vi "Convert I2C Messages & Buffer.vi"(8 "error in (no error)":errorcluster, 11 "Data":u8[](array[numeric])) -> (0 "error out":errorcluster)   [LabVIEW 2025, in "I2C Bus Monitor UI.lvlib"]
uses:
  I2C Bus Monitor UI.lvlib
  Table Buffer - Enqueue.vi
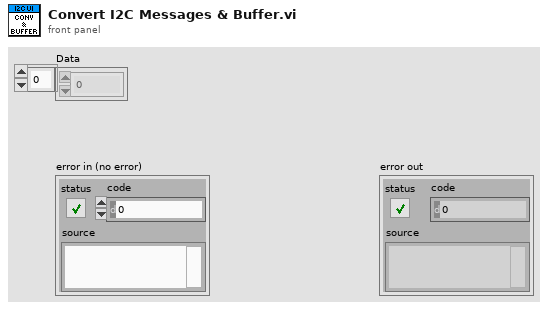
[diagram p1: front panel]
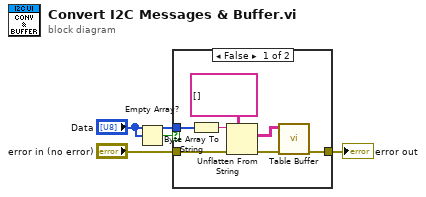
[diagram p0: block diagram]
diagram:
  n1 = Empty Array?(array="Data") -> (empty?=w2:bool)
  n2 = case shown="False" w2 {
    tunnel: "error in (no error)" -> [w6 w12]
    tunnel: "Data" -> [w9 _]
    tunnel: [w7 w12] -> w4
    frame False {
      n3 = Byte Array To String(unsigned byte array=w9) -> (string=w10:string)
      n4 = Unflatten From String(type=string[][] [] ("Fetched I2C Messages"), binary string=w10, error in (no error)=w6) -> (value=w5:string[][], error out=w8:errorcluster)  [unwired: 2 in, 1 out]
      n5 = call-poly "Table Buffer.vi"("error in (no error)"=w8, "Data"=w5) -> ("error out"=w7:errorcluster)  [unwired: 9 in]
    }
    frame True {
    }
  }
  "error out" <- w4
